vi "Parse Member.vi"(8 "error in (no error)":errorcluster, 10 "member":string, 11 "Subscription in":refnum<class "Subscription.lvclass">) -> (0 "error out":errorcluster, 3 "Subscription out":refnum<class "Subscription.lvclass">)   [LabVIEW 2015, in "NI_AWS_SNS.lvlib" / "Subscription.lvclass"]
uses:
  Subscription.lvclass
  Subscription Protocol.ctl
  Subscription.lvclass/Subscription.ctl
  Write Endpoint.vi
  Write Owner.vi
  Write Protocol.vi
  Write Topic.vi
  Core/ARN/ARN.lvclass
  Core/HTTP Request/HTTP Request.lvclass
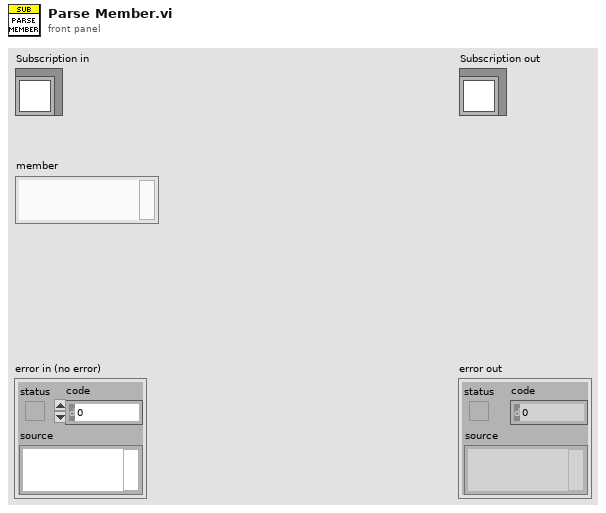
[diagram p1: front panel]
types:
  T1 = typedef "NI_AWS_SNS.lvlib/Subscription.lvclass/Subscription Protocol.ctl" = enum16{"http", "https", "email", "email-json", "sms", "sqs", "application", "lambda"}
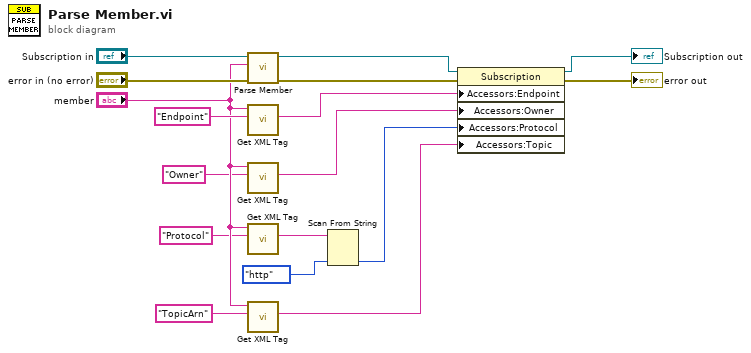
[diagram p0: block diagram]
diagram:
  n1 = call-parent "Parse Member.vi"("error in (no error)"="error in (no error)", "member"="member", "ARN in"="Subscription in") -> ("error out"=w13:errorcluster, "ARN out"=w15:refnum<class "Subscription.lvclass">)  [unwired: 7 in]
  n2 = call "Get XML Tag.vi"("Tag name"="Endpoint", "XML String in"="member") -> ("Tag value"=w10:string)  [unwired: 5 in, 4 out]
  n3 = call "Get XML Tag.vi"("Tag name"="Owner" ("XML String in"), "XML String in"="member") -> ("Tag value"=w8:string)  [unwired: 5 in, 4 out]
  n4 = call "Get XML Tag.vi"("Tag name"="Protocol" ("XML String in"), "XML String in"="member") -> ("Tag value"=w9:string)  [unwired: 5 in, 4 out]
  n5 = call "Get XML Tag.vi"("Tag name"="TopicArn" ("XML String in"), "XML String in"="member") -> ("Tag value"=w5:string)  [unwired: 5 in, 4 out]
  n6 = Scan From String(input string=w9, default 1=Subscription_Protocol."http" ("Subscription Protocol")) -> (output 1=w6:T1)  [unwired: 3 in, 3 out]
  n7 = property class="Subscription"(reference=w15, error in=w13, "Accessors:Endpoint"=w10, "Accessors:Owner"=w8, "Accessors:Protocol"=w6, "Accessors:Topic"=w5) -> (reference out=→"Subscription out":refnum<class "Subscription.lvclass">, error out=→"error out":errorcluster)
